vi "Set FPGA Reference.vi"(8 "Error In":errorcluster, 10 "FPGA Reference":T1, 11 "Draw Frame In":refnum<class "Draw Frame.lvclass">) -> (0 "Error Out":errorcluster, 3 "Draw Frame Out":refnum<class "Draw Frame.lvclass">)   [LabVIEW 2019, in "Draw Frame.lvclass"]
uses:
  Draw Frame.lvclass
  Public/Controls/FPGA Reference.ctl
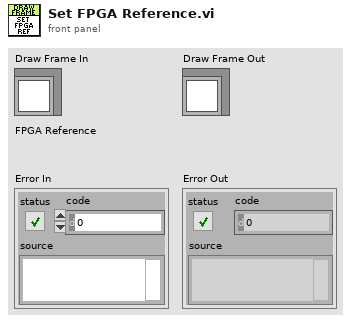
[diagram p1: front panel]
types:
  T1 = typedef "Draw Frame.lvclass/FPGA Reference.ctl" = refnum<k20>
  T2 = typedef "Draw Frame.lvclass/Data.ctl" = cluster{"Display":refnum<class "Display.lvclass">, "FPGA Reference":T1}
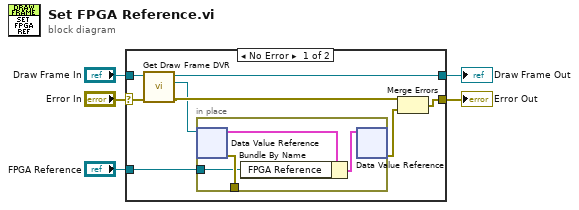
[diagram p0: block diagram]
diagram:
  n1 = case shown="No Error" "Error In" {
    selector: "Error In" -> [w10 w18]
    tunnel: [w12 w18] -> w2
    tunnel: [w9 w19] -> w5
    tunnel: "Draw Frame In" -> [w11 w19]
    tunnel: "FPGA Reference" -> [w6 _]
    frame No Error {
      n2 = call "Get Draw Frame DVR.vi"("Error In"=w10, "Draw Frame In"=w11) -> ("Error Out"=w8:errorcluster, "DVR"=w7:refnum<data-value>, "Draw Frame Out"=w9:refnum<class "Draw Frame.lvclass">)  [unwired: 7 in]
      n3 = in-place {
        in-place-border: [w17] -> _
        in-place-border: w6 -> [w14]
        n4 = in-place-dvr #1(w7) -> (w16:T2, w17:errorcluster)
        n5 = Bundle By Name(cluster=w16, "FPGA Reference"=w14) -> (w15:T2)
        n6 = in-place-dvr #1(w15) -> (w13:errorcluster)  [unwired: 1 out]
      }
      n7 = Merge Errors(w8, w13) -> (w12:errorcluster)
    }
    frame Error {
    }
  }
  "Draw Frame Out" <- w5
  "Error Out" <- w2
